vi "Calculate ROI.vi"(0 "image in":refnum<class "MSC Image.lvclass">, 1 "ROIs In":T1[](array[typedef]) {"Type" items=["Point", "Line", "Rectangle", "Oval", "Freehand / Polygon"]}, 2 "ROI ID":i32, 5 "error in (no error)":errorcluster, 8 "Keep images?":bool) -> (14 "image out":refnum<class "MSC Image.lvclass">, 15 "ROI":T1 {"Type" items=["Point", "Line", "Rectangle", "Oval", "Freehand / Polygon"]}, 16 "particle image out":refnum<class "MSC Image.lvclass">, 17 "particle mask image out":refnum<class "MSC Image.lvclass">, 19 "error out":errorcluster)   [LabVIEW 2016, in "MSC Image.lvclass"]
doc: "Lowlevel ROI calculation vi."
uses:
  MSC Image.lvclass
  controls/Contour.ctl
  controls/ROI Type.ctl
  controls/Contour hierarchy.ctl
  controls/ROI.ctl
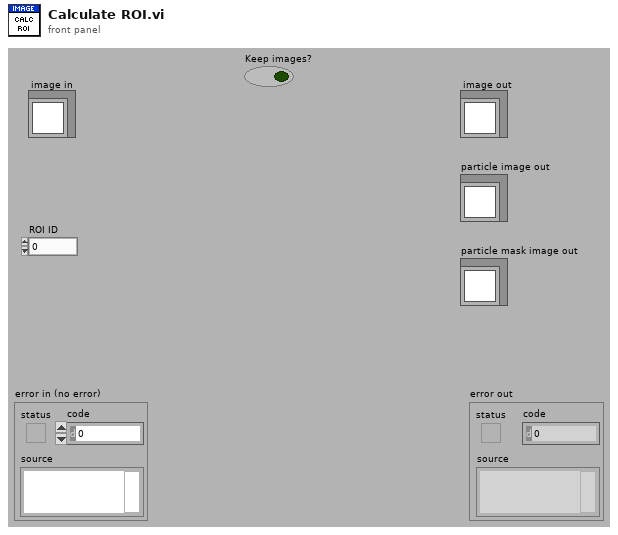
[diagram p1: front panel]
types:
  T1 = typedef "MSC Image.lvclass/ROI.ctl" = cluster{"Type":T2, "Parameters":dbl[], "Contour":T3, "Bounding Box":T3, "Contour Length":dbl, "ROI Area":dbl, "ROI Mean":dbl, "ROI Standard Deviation":dbl, "ROI Min":dbl, "ROI Max":dbl, "Hierarchy":T4, "Variant":variant, "Timestamp":timestamp}
  T2 = typedef "MSC Image.lvclass/ROI Type.ctl" = u16
  T3 = typedef "MSC Image.lvclass/Contour.ctl" = cluster{"x":i16, "y":i16}[]
  T4 = typedef "MSC Image.lvclass/Contour hierarchy.ctl" = cluster{"parent ID":i32, "children IDs":dbl[], "level":i32}
  T5 = typedef "MSC Image.lvclass/Size.ctl" = cluster{"Cols":i32, "Rows":i32}
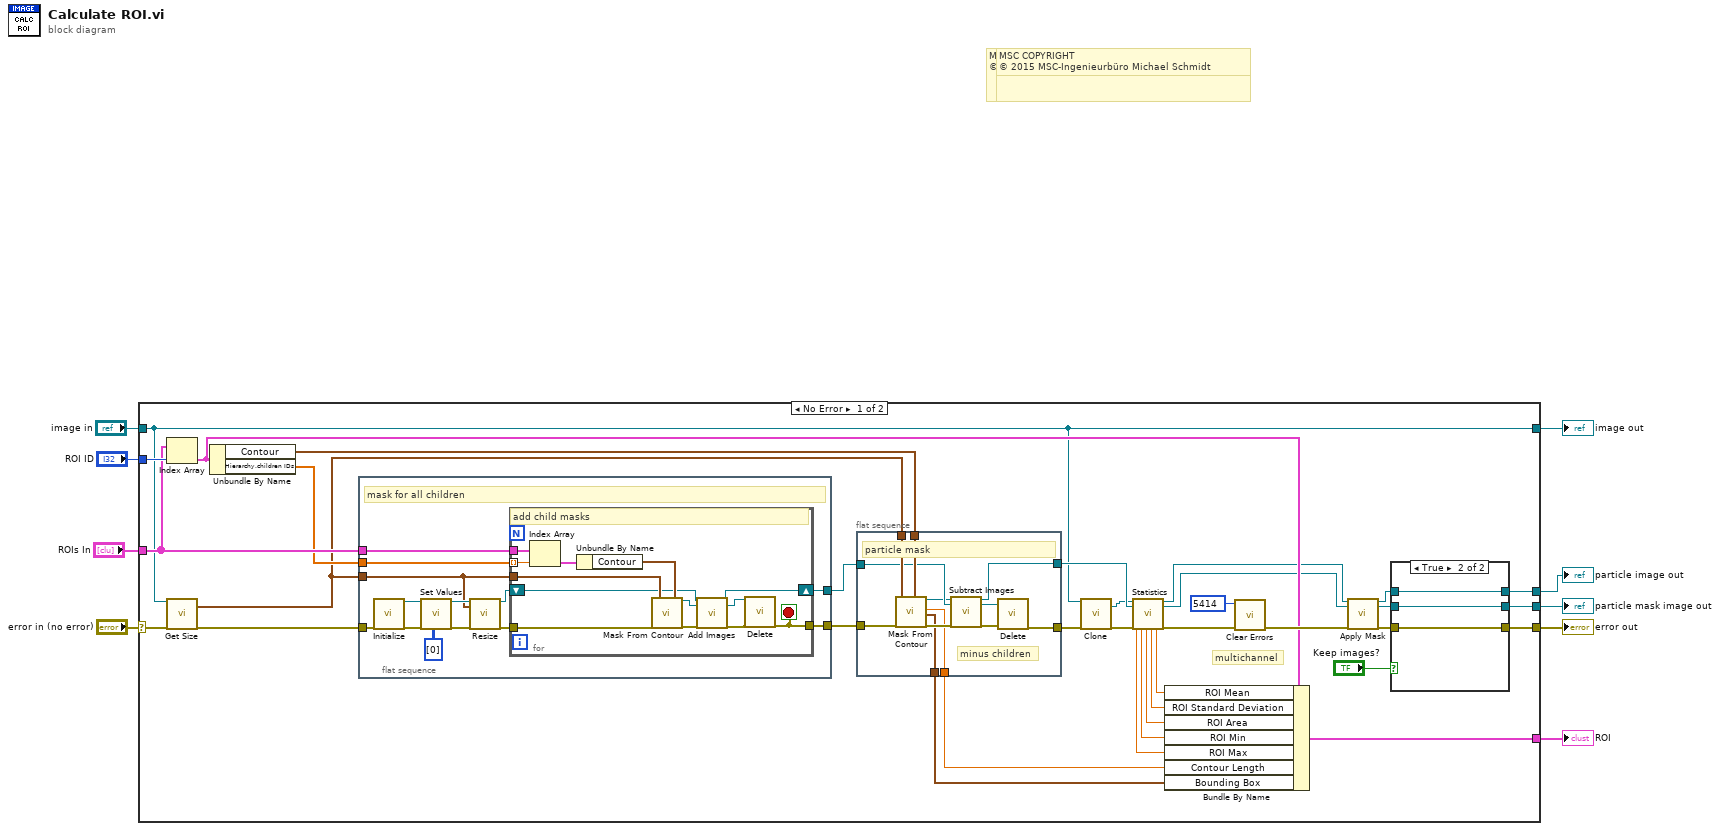
[diagram p0: block diagram]
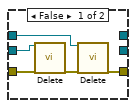
[diagram p2: hidden frame]
diagram:
  # "MSC COPYRIGHT\n© 2016 MSC-Ingenieurbüro Michael Schmidt"
  # "MSC COPYRIGHT\n© 2016 MSC-Ingenieurbüro Michael Schmidt"
  # "MSC COPYRIGHT\n© 2015 MSC-Ingenieurbüro Michael Schmidt"
  # "MSC COPYRIGHT\n© 2015 MSC-Ingenieurbüro Michael Schmidt"
  n1 = case shown="No Error" "error in (no error)" {
    selector: "error in (no error)" -> [w44 w92]
    tunnel: [w27 w92] -> w8
    tunnel: [w13 w91] -> w6
    tunnel: "image in" -> [w13 w91]
    tunnel: "ROIs In" -> [w42 _]
    tunnel: "ROI ID" -> [w43 _]
    tunnel: [w26 _] -> w3
    tunnel: [w25 _] -> w2
    tunnel: [w15 _] -> w1
    frame No Error {
      # "multichannel"
      n2 = Index Array(array=w42, index=w43) -> (element=w24:T1)
      n3 = call-dynamic "Get Size.vi"("image in"=w13, "error in (no error)"=w44) -> ("Size"=w37:T5, "error out"=w40:errorcluster)  [unwired: 15 in, 1 out]
      n4 = Unbundle By Name(w24) -> ("Contour"=w38:T3, "Hierarchy.children IDs"=w41:dbl[])
      n5 = flat-sequence {
        tunnel: w41 -> [w77]
        tunnel: w42 -> [w76]
        tunnel: w40 -> [w75]
        tunnel: w37 -> [w67]
        tunnel: [w66] -> w39
        tunnel: [w65] -> w36
        frame #0 {
          # "mask for all children"
          n6 = call "Initialize.vi"("error in (no error)"=w75) -> ("image out"=w72:refnum<class "MSC Image.lvclass">, "error out"=w73:errorcluster)  [unwired: 17 in]
          n7 = call-dynamic "Set Values.vi"("image in"=w72, "imageData U8"=u8[][] [[0]], "error in (no error)"=w73) -> ("image out"=w70:refnum<class "MSC Image.lvclass">, "error out"=w71:errorcluster)  [unwired: 15 in]
          n8 = call-dynamic "Resize.vi"("image in"=w70, "Size"=w67, "error in (no error)"=w71) -> ("image out"=w69:refnum<class "MSC Image.lvclass">, "error out"=w68:errorcluster)  [unwired: 15 in]
          n9 = for {
            tunnel: w76 -> [w90]
            tunnel: w77 -> [w88] mode=indexing
            shift-right: [w79] -> w65
            shift-left: w69 -> [w83]
            tunnel: w68 -> [w85]
            tunnel: w67 -> [w87]
            tunnel: [w78] -> w66
            stop <- w78 stop-if-true
            # "add child masks"
            n10 = Index Array(array=w90, index=w88) -> (element=w89:T1)
            n11 = Unbundle By Name(w89) -> ("Contour"=w86:T3)
            n12 = call "Mask From Contour.vi"("Contour"=w86, "Size"=w87, "error in (no error)"=w85) -> ("image out"=w82:refnum<class "MSC Image.lvclass">, "error out"=w84:errorcluster)  [unwired: 12 in, 3 out]
            n13 = call-dynamic "Add Images.vi"("image in"=w83, "image 2 in"=w82, "error in (no error)"=w84) -> ("image out"=w79:refnum<class "MSC Image.lvclass">, "image 2 out"=w81:refnum<class "MSC Image.lvclass">, "error out"=w80:errorcluster)  [unwired: 14 in]
            n14 = call-dynamic "Delete.vi"("image in"=w81, "error in (no error)"=w80) -> ("error out"=w78:errorcluster)  [unwired: 17 in]
          }
        }
      }
      n15 = flat-sequence {
        tunnel: w39 -> [w64]
        tunnel: w38 -> [w63]
        tunnel: w37 -> [w62]
        tunnel: w36 -> [w54]
        tunnel: [w58] -> w35
        tunnel: [w57] -> w14
        tunnel: [w56] -> w17
        tunnel: [w55] -> w16
        frame #0 {
          # "minus children"
          # "particle mask"
          n16 = call "Mask From Contour.vi"("Contour"=w63, "Size"=w62, "error in (no error)"=w64) -> ("image out"=w53:refnum<class "MSC Image.lvclass">, "contourLengthPixel"=w55:dbl, "Bounding Box"=w56:T3, "error out"=w61:errorcluster)  [unwired: 12 in, 1 out]
          n17 = call-dynamic "Subtract Images.vi"("image in"=w53, "image 2 in"=w54, "error in (no error)"=w61) -> ("image out"=w57:refnum<class "MSC Image.lvclass">, "image 2 out"=w60:refnum<class "MSC Image.lvclass">, "error out"=w59:errorcluster)  [unwired: 14 in]
          n18 = call-dynamic "Delete.vi"("image in"=w60, "error in (no error)"=w59) -> ("error out"=w58:errorcluster)  [unwired: 17 in]
        }
      }
      n19 = call-dynamic "Clone.vi"("image in"=w13, "error in (no error)"=w35) -> ("clone image out"=w10:refnum<class "MSC Image.lvclass">, "error out"=w20:errorcluster)  [unwired: 15 in, 1 out]
      n20 = call-dynamic "Statistics.vi"("image in"=w10, "mask image in"=w14, "error in (no error)"=w20) -> ("mean"=w23:dbl, "stdDev"=w22:dbl, "area"=w21:dbl, "image out"=w12:refnum<class "MSC Image.lvclass">, "mask image out"=w11:refnum<class "MSC Image.lvclass">, "min"=w19:dbl, "max"=w18:dbl, "error out"=w33:errorcluster)  [unwired: 9 in]
      n21 = Bundle By Name(cluster=w24, "ROI Mean"=w23, "ROI Standard Deviation"=w22, "ROI Area"=w21, "ROI Min"=w19, "ROI Max"=w18, "Contour Length"=w16, "Bounding Box"=w17) -> (w15:T1)
      n22 = call <vilib>:"Clear Errors.vi"("error in (no error)"=w33, "specific error code to clear (0: all)"=5414 ("code")) -> ("error out"=w29:errorcluster)  [unwired: 4 in, 1 out]
      n23 = call-dynamic "Apply Mask.vi"("image in"=w12, "mask image in"=w11, "error in (no error)"=w29) -> ("image out"=w30:refnum<class "MSC Image.lvclass">, "mask image out"=w31:refnum<class "MSC Image.lvclass">, "error out"=w28:errorcluster)  [unwired: 14 in]
      n24 = case shown="True" "Keep images?" {
        tunnel: w31 -> [w49 w52]
        tunnel: w30 -> [w48 w50]
        tunnel: w28 -> [w47 w51]
        tunnel: [w45 w51] -> w27
        tunnel: [_ w52] -> w25
        tunnel: [_ w50] -> w26
        frame False {
          n25 = call-dynamic "Delete.vi"("image in"=w49, "error in (no error)"=w47) -> ("error out"=w46:errorcluster)  [unwired: 17 in]
          n26 = call-dynamic "Delete.vi"("image in"=w48, "error in (no error)"=w46) -> ("error out"=w45:errorcluster)  [unwired: 17 in]
        }
        frame True {
        }
      }
    }
    frame Error {
    }
  }
  "error out" <- w8
  "image out" <- w6
  "particle image out" <- w3
  "particle mask image out" <- w2
  "ROI" <- w1
